vi "Acquire Infrared Image.vi"() -> ()   [LabVIEW 2014, in "LVH-KinectOne.lvlib"]
uses:
  LVH-KinectOne.lvlib
  Private/kinectRead [Infrared Frame].vi
panel:
  out "Infrared Image":T1(plugin-control)
  in  "stop":bool
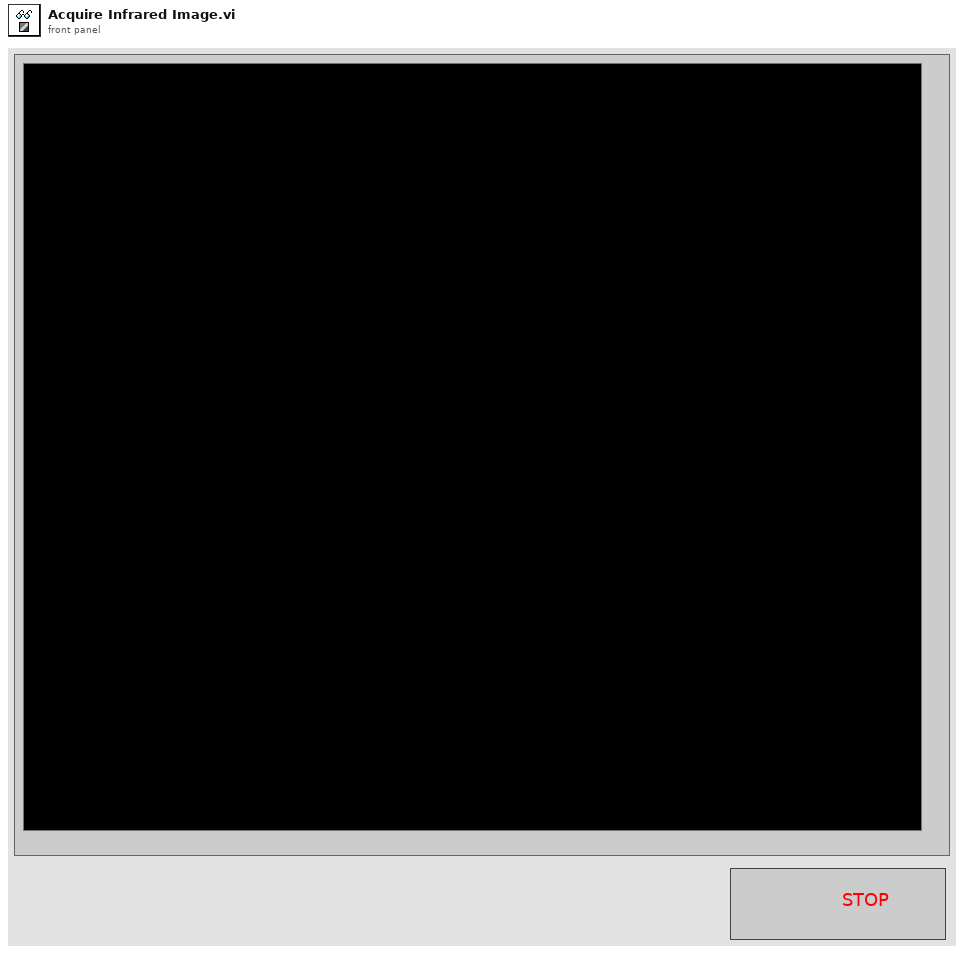
[diagram p1: front panel]
types:
  T1 = typedef "IMAQ Image.ctl" = refnum<image>
  T2 = typedef "Image Type" = u32
  T3 = typedef "LVH-KinectOne.lvlib/KinectSensor References.ctl" = cluster{"KinectSensor":refnum<k24>, "MultiSourceFrameReader":refnum<k24>, "BodyFrameDataInterface":refnum<k24>}
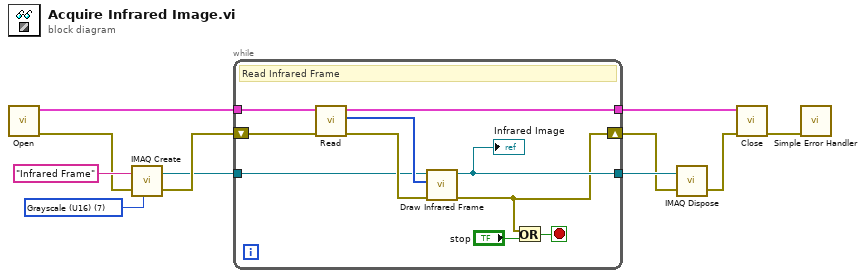
[diagram p0: block diagram]
diagram:
  w10 = T2 7 items=["Grayscale (U8)", "Grayscale (I16)", "Grayscale (SGL)", "Complex (CSG)", "RGB (U32)", "HSL (U32)", "RGB (U64)", "Grayscale (U16)"] ("Image Type")
  n1 = call "Open.vi"() -> ("error out"=w2:errorcluster, "KinectSensor References out"=w1:T3)  [unwired: 10 in]
  n2 = call "IMAQ Create"("Image Name"="Infrared Frame", "Image Type"=w10, "error in (no error)"=w2) -> ("New Image"=w8:T1, "error out"=w9:errorcluster)  [unwired: 2 in]
  n3 = while {
    tunnel: w1 -> [w21]
    tunnel: [w17] -> w11
    shift-right: [w13] -> w6
    shift-left: w9 -> [w20]
    tunnel: w8 -> [w16]
    tunnel: [w15] -> w7
    stop <- w12 stop-if-true
    # "Read Infrared Frame"
    n4 = call-poly "Read.vi"("error in (no error)"=w20, "KinectSensor References in"=w21) -> ("error out"=w19:errorcluster, "frameData"=w18:u16[], "KinectSensor References out"=w17:T3)  [unwired: 7 in]
    n5 = call "Draw Infrared Frame.vi"("error in (no error)"=w19, "U16 Array"=w18, "Image"=w16) -> ("error out"=w13:errorcluster, "Image Out"=w15:T1)  [unwired: 7 in]
    "Infrared Image" <- w15
    n6 = Or(x=w13, y="stop") -> (x .or. y?=w12:bool)
  }
  n7 = call "IMAQ Dispose"("Image"=w7, "error in (no error)"=w6) -> ("error out"=w5:errorcluster)  [unwired: 4 in]
  n8 = call "Close.vi"("error in"=w5, "KinectSensor References"=w11) -> ("error out"=w3:errorcluster)  [unwired: 9 in]
  n9 = call <vilib>:"Simple Error Handler.vi"("error in (no error)"=w3) -> ()  [unwired: 4 in, 5 out]
